vi "AI SetAverage.vi"(4 "error in":errorcluster, 6 "Number to average":i32=100, 7 "params in":T1={"Manual Control"={"Rotation Control"={"Phase"=0.0, "A amp (0-120)"=75.0, "B amp (0-120)"=53.3, "mean freq  [MHz]\ndefault 39.99"=40.0, "freq difference [Hz]"=2.0, "Enable A"=TRUE, "Enable B"=TRUE}, "X piezo\n [nm]"=0.0, "Y peizo\n [nm]"=0.0, "-Z piezo\n [nm]"=5.012658227848101, "AOM0 \nPower"=0.2}, "Piezo Calibr"={"Px2Vx(AO)"=nan, "Py2Vy(AO)"=nan, "Pz2Vz(AO)"=nan, "Min Px"=nan, "Min Py"=nan, "Min Pz"=nan, "Max Px"=nan, "Max Py"=nan, "Max Pz"=nan, "Vx0 (V)"=nan, "Vy0 (V)"=nan, "Vz0 (V)"=nan}, "Instrument Calibr"={"Angular compensation coeffs"=[], "TetherCenter"={"TrapX_AO 0 [nm]"=nan, "TrapY_AO 0 [nm]"=nan, "TrapZ_AO 0 [nm]"=nan}, "XYZsignal baseline"={"Xsignal0"=nan, "Ysignal0"=nan, "Zsignal0"=nan, "Zsig slope"=nan, "Z bead0"=nan}, "S and P to Vs0"={"Vs0/P"=1.0, "Vs0/S"=1.0}, "Psi"=0.0, "ePS:eRL drift correlation"={"Interc P"=nan, "Slope P"=nan, "Interc S"=nan, "Slope S"=nan}, "Current piezo volt AO"={"Vpx_AO [V]"=nan, "Vpy_AO [V]"=nan, "Vpz_AO [V]"=nan}}, "Cylinder Calibr"={"ZStiff"=nan, "Zsens"=nan, "AngStiff"=nan, "XStiff"=nan, "Xsens"=nan, "MaxEllip"=nan, "YStiff"=nan, "Ysens"=nan, "FocalShift"=nan, "Sfz"=nan, "1/Sz"=nan, "Stau"=nan, "Sfx"=nan, "1/Sx"=nan, "1/Sang"=nan, "Sfy"=nan, "1/Sy"=nan, "1/focal"=nan}, "DAQParams"={"Buffer size"=nan, "Scanning rate"=nan, "Average"=nan, "Sampling rate"=nan, "set dt"=nan}, "DAQ channel offsets"={"A0 [V]"=0.0, "D0 [V]"=0.0, "P0  [V]"=0.0, "S0 [V]"=0.0, "L0 [V]"=0.0, "R0 [V]"=0.0, "Vpx0 [V]"=0.0, "Vpy0 [V]"=0.0, "Vpz0 [V]"=0.0, "Vsum0 [V]"=0.0, "Vpx_AO0 [V]"=0.0, "Vpy_AO0 [V]"=0.0, "Vpz_AO0 [V]"=0.0}, "Z bead polynomial coeffs"=[nan, nan, nan, nan], "Skip button ref"=refnum, "z bead lookup table"={"z signal"=[], "z bead"=[]}, "SP->power Matrix"=[], "Ms2p"=[], "Mp2s"=[], "Polynomial coeff V_px,y,z 2 position (nm)"=[], "task in"=""} {"Instrument Calibr"."Psi" format="%#_2f"; "Manual Control"."Y peizo\n [nm]" scale=0.0..7000.0; "Manual Control"."AOM0 \nPower" scale=0.0..1.0; "Manual Control"."X piezo\n [nm]" scale=0.0..7000.0; "Manual Control"."Rotation Control"."freq difference [Hz]" step=0.5; "Manual Control"."Rotation Control"."mean freq  [MHz]\ndefault 39.99" min=0.0 step=0.01; "Manual Control"."Rotation Control"."B amp (0-120)" min=0.0 max=120.0 step=0.1; "Manual Control"."Rotation Control"."A amp (0-120)" min=0.0 max=120.0 step=0.1; "Manual Control"."Rotation Control"."Phase" scale=0.0..360.0; "Manual Control"."-Z piezo\n [nm]" scale=1000.0..7000.0}) -> (0 "error out":errorcluster, 3 "params out":T1={"Manual Control"={"Rotation Control"={"Phase"=0.0, "A amp (0-120)"=75.0, "B amp (0-120)"=53.3, "mean freq  [MHz]\ndefault 39.99"=40.0, "freq difference [Hz]"=2.0, "Enable A"=TRUE, "Enable B"=TRUE}, "X piezo\n [nm]"=0.0, "Y peizo\n [nm]"=0.0, "-Z piezo\n [nm]"=5.012658227848101, "AOM0 \nPower"=0.2}, "Piezo Calibr"={"Px2Vx(AO)"=nan, "Py2Vy(AO)"=nan, "Pz2Vz(AO)"=nan, "Min Px"=nan, "Min Py"=nan, "Min Pz"=nan, "Max Px"=nan, "Max Py"=nan, "Max Pz"=nan, "Vx0 (V)"=nan, "Vy0 (V)"=nan, "Vz0 (V)"=nan}, "Instrument Calibr"={"Angular compensation coeffs"=[], "TetherCenter"={"TrapX_AO 0 [nm]"=nan, "TrapY_AO 0 [nm]"=nan, "TrapZ_AO 0 [nm]"=nan}, "XYZsignal baseline"={"Xsignal0"=nan, "Ysignal0"=nan, "Zsignal0"=nan, "Zsig slope"=nan, "Z bead0"=nan}, "S and P to Vs0"={"Vs0/P"=1.0, "Vs0/S"=1.0}, "Psi"=0.0, "ePS:eRL drift correlation"={"Interc P"=nan, "Slope P"=nan, "Interc S"=nan, "Slope S"=nan}, "Current piezo volt AO"={"Vpx_AO [V]"=nan, "Vpy_AO [V]"=nan, "Vpz_AO [V]"=nan}}, "Cylinder Calibr"={"ZStiff"=nan, "Zsens"=nan, "AngStiff"=nan, "XStiff"=nan, "Xsens"=nan, "MaxEllip"=nan, "YStiff"=nan, "Ysens"=nan, "FocalShift"=nan, "Sfz"=nan, "1/Sz"=nan, "Stau"=nan, "Sfx"=nan, "1/Sx"=nan, "1/Sang"=nan, "Sfy"=nan, "1/Sy"=nan, "1/focal"=nan}, "DAQParams"={"Buffer size"=nan, "Scanning rate"=nan, "Average"=nan, "Sampling rate"=nan, "set dt"=nan}, "DAQ channel offsets"={"A0 [V]"=0.0, "D0 [V]"=0.0, "P0  [V]"=0.0, "S0 [V]"=0.0, "L0 [V]"=0.0, "R0 [V]"=0.0, "Vpx0 [V]"=0.0, "Vpy0 [V]"=0.0, "Vpz0 [V]"=0.0, "Vsum0 [V]"=0.0, "Vpx_AO0 [V]"=0.0, "Vpy_AO0 [V]"=0.0, "Vpz_AO0 [V]"=0.0}, "Z bead polynomial coeffs"=[nan, nan, nan, nan], "Skip button ref"=refnum, "z bead lookup table"={"z signal"=[], "z bead"=[]}, "SP->power Matrix"=[], "Ms2p"=[], "Mp2s"=[], "Polynomial coeff V_px,y,z 2 position (nm)"=[], "task in"=""} {"Instrument Calibr"."Psi" format="%#_2f"; "Manual Control"."Y peizo\n [nm]" scale=0.0..7000.0; "Manual Control"."AOM0 \nPower" scale=0.0..1.0; "Manual Control"."X piezo\n [nm]" scale=0.0..7000.0; "Manual Control"."Rotation Control"."freq difference [Hz]" step=0.5; "Manual Control"."Rotation Control"."mean freq  [MHz]\ndefault 39.99" min=0.0 step=0.01; "Manual Control"."Rotation Control"."B amp (0-120)" min=0.0 max=120.0 step=0.1; "Manual Control"."Rotation Control"."A amp (0-120)" min=0.0 max=120.0 step=0.1; "Manual Control"."Rotation Control"."Phase" scale=0.0..360.0; "Manual Control"."-Z piezo\n [nm]" scale=1000.0..7000.0})   [LabVIEW 2017, in "Data aquisition.lvlib"]
uses:
  Data aquisition.lvlib
  Initialization/New Param_170907.ctl
  Initialization/ManualCtrl.ctl
  Initialization/CylinderCalibrNew.ctl
  SignalConversion/DAQChannelOffsets.ctl
  <vilib>/Analysis/Matrix/Datatypes/RealMatrix.ctl
  Initialization/Initialization.lvlib
  <vilib>/Analysis/Matrix/NI_Matrix.lvlib
  SignalConversion/SignalConverson.lvlib
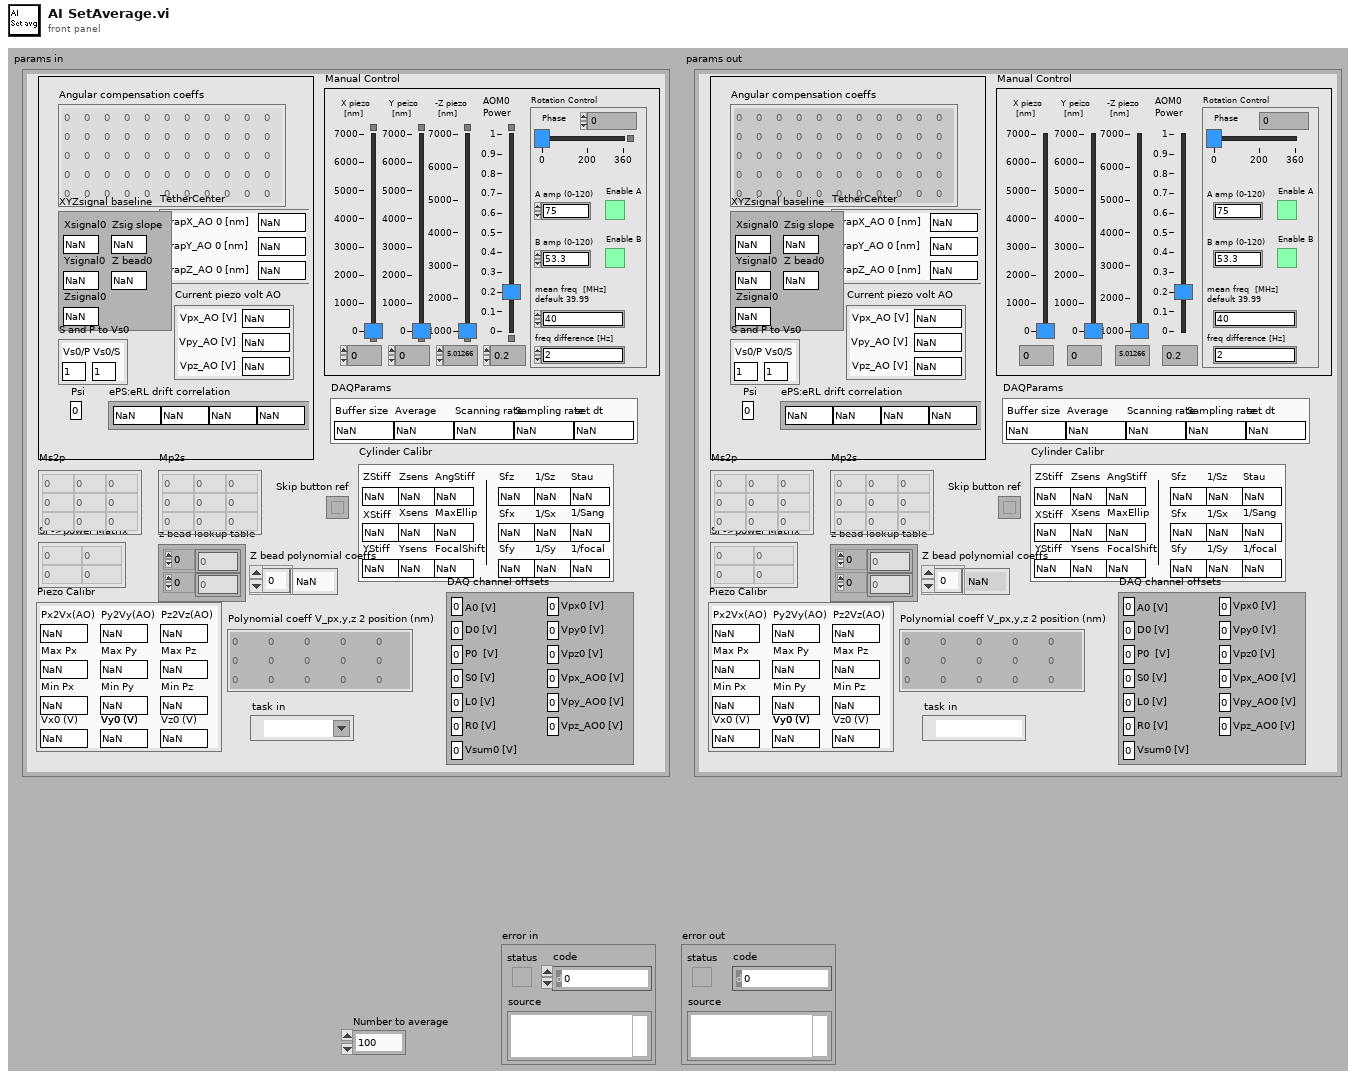
[diagram p1: front panel]
types:
  T1 = typedef "Initialization.lvlib/New Param_170907.ctl" = cluster{"Manual Control":T2, "Piezo Calibr":cluster{"Px2Vx(AO)":dbl, "Py2Vy(AO)":dbl, "Pz2Vz(AO)":dbl, "Min Px":dbl, "Min Py":dbl, "Min Pz":dbl, "Max Px":dbl, "Max Py":dbl, "Max Pz":dbl, "Vx0 (V)":dbl, "Vy0 (V)":dbl, "Vz0 (V)":dbl}, "Instrument Calibr":cluster{"Angular compensation coeffs":dbl[][], "TetherCenter":cluster{"TrapX_AO 0 [nm]":dbl, "TrapY_AO 0 [nm]":dbl, "TrapZ_AO 0 [nm]":dbl}, "XYZsignal baseline":cluster{"Xsignal0":dbl, "Ysignal0":dbl, "Zsignal0":dbl, "Zsig slope":dbl, "Z bead0":dbl}, "S and P to Vs0":cluster{"Vs0/P":dbl, "Vs0/S":dbl}, "Psi":dbl, "ePS:eRL drift correlation":cluster{"Interc P":dbl, "Slope P":dbl, "Interc S":dbl, "Slope S":dbl}, "Current piezo volt AO":cluster{"Vpx_AO [V]":dbl, "Vpy_AO [V]":dbl, "Vpz_AO [V]":dbl}}, "Cylinder Calibr":T3, "DAQParams":cluster{"Buffer size":dbl, "Scanning rate":dbl, "Average":dbl, "Sampling rate":dbl, "set dt":dbl}, "DAQ channel offsets":T4, "Z bead polynomial coeffs":dbl[], "Skip button ref":refnum<vi>, "z bead lookup table":cluster{"z signal":dbl[], "z bead":dbl[]}, "SP->power Matrix":T5, "Ms2p":T5, "Mp2s":T5, "Polynomial coeff V_px,y,z 2 position (nm)":dbl[][], "task in":refnum<k21>}
  T2 = typedef "Initialization.lvlib/ManualCtrl.ctl" = cluster{"Rotation Control":cluster{"Phase":dbl, "A amp (0-120)":dbl, "B amp (0-120)":dbl, "mean freq  [MHz]\ndefault 39.99":dbl, "freq difference [Hz]":dbl, "Enable A":bool, "Enable B":bool}, "X piezo\n [nm]":dbl, "Y peizo\n [nm]":dbl, "-Z piezo\n [nm]":dbl, "AOM0 \nPower":dbl}
  T3 = typedef "Initialization.lvlib/CylinderCalibrNew.ctl" = cluster{"ZStiff":dbl, "Zsens":dbl, "AngStiff":dbl, "XStiff":dbl, "Xsens":dbl, "MaxEllip":dbl, "YStiff":dbl, "Ysens":dbl, "FocalShift":dbl, "Sfz":dbl, "1/Sz":dbl, "Stau":dbl, "Sfx":dbl, "1/Sx":dbl, "1/Sang":dbl, "Sfy":dbl, "1/Sy":dbl, "1/focal":dbl}
  T4 = typedef "SignalConverson.lvlib/DAQChannelOffsets.ctl" = cluster{"A0 [V]":dbl, "D0 [V]":dbl, "P0  [V]":dbl, "S0 [V]":dbl, "L0 [V]":dbl, "R0 [V]":dbl, "Vpx0 [V]":dbl, "Vpy0 [V]":dbl, "Vpz0 [V]":dbl, "Vsum0 [V]":dbl, "Vpx_AO0 [V]":dbl, "Vpy_AO0 [V]":dbl, "Vpz_AO0 [V]":dbl}
  T5 = typedef "NI_Matrix.lvlib/RealMatrix.ctl" = dbl[][]
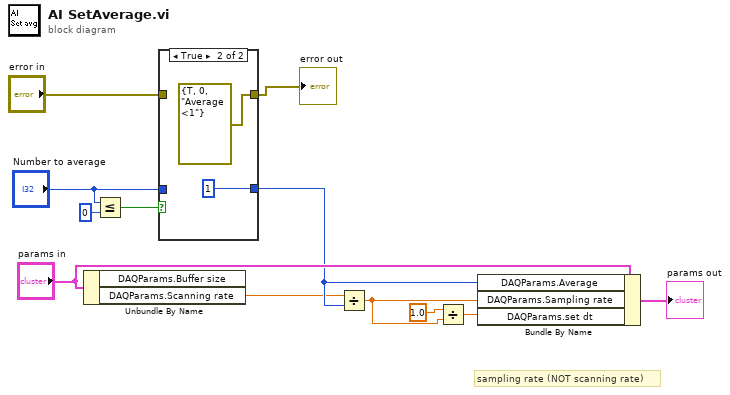
[diagram p0: block diagram]
diagram:
  # "sampling rate (NOT scanning rate)"
  n1 = Unbundle By Name("params in") -> ("DAQParams.Scanning rate"=w2:dbl)  [unwired: 1 out]
  n2 = Less Or Equal?(x="Number to average", y=0) -> (x <= y?=w9:bool)
  n3 = case shown="True" w9 {
    tunnel: [w14 1] -> w3
    tunnel: "Number to average" -> [w14 _]
    tunnel: "error in" -> [w13 _]
    tunnel: [w13 errorcluster {"status"=TRUE, "code"=0, "source"="Average <1"} ("error in")] -> w1
    frame False {
    }
    frame True {
    }
  }
  "error out" <- w1
  n4 = Divide(x=w2, y=w3) -> (x/y=w4:dbl)
  n5 = Divide(x=1.0, y=w4) -> (x/y=w6:dbl)
  n6 = Bundle By Name(cluster="params in", "DAQParams.Average"=w3, "DAQParams.Sampling rate"=w4, "DAQParams.set dt"=w6) -> (→"params out":T1)
